vi "HB_ReadAIAllChannels.vi"(8 "error in (no error)":errorcluster, 11 "HBDeviceRef":T1) -> (0 "error out":errorcluster, 1 "All Channels Raw Values":u32[](array[numeric]) format="%012b", 2 "All Channels Scaled Values":dbl[](array[numeric]), 3 "HBDeviceRef":T1)   [LabVIEW 2016]
uses:
  <vilib>/Rock Robotics/WPI/SerialPort/WPI_SerialPortRef.ctl
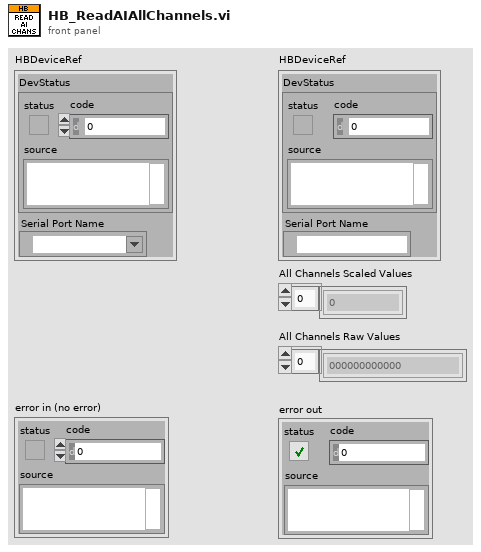
[diagram p1: front panel]
types:
  T1 = typedef "WPI_SerialPortRef.ctl" = cluster{"DevStatus":errorcluster, "Serial Port Name":refnum<visa-resource-name>}
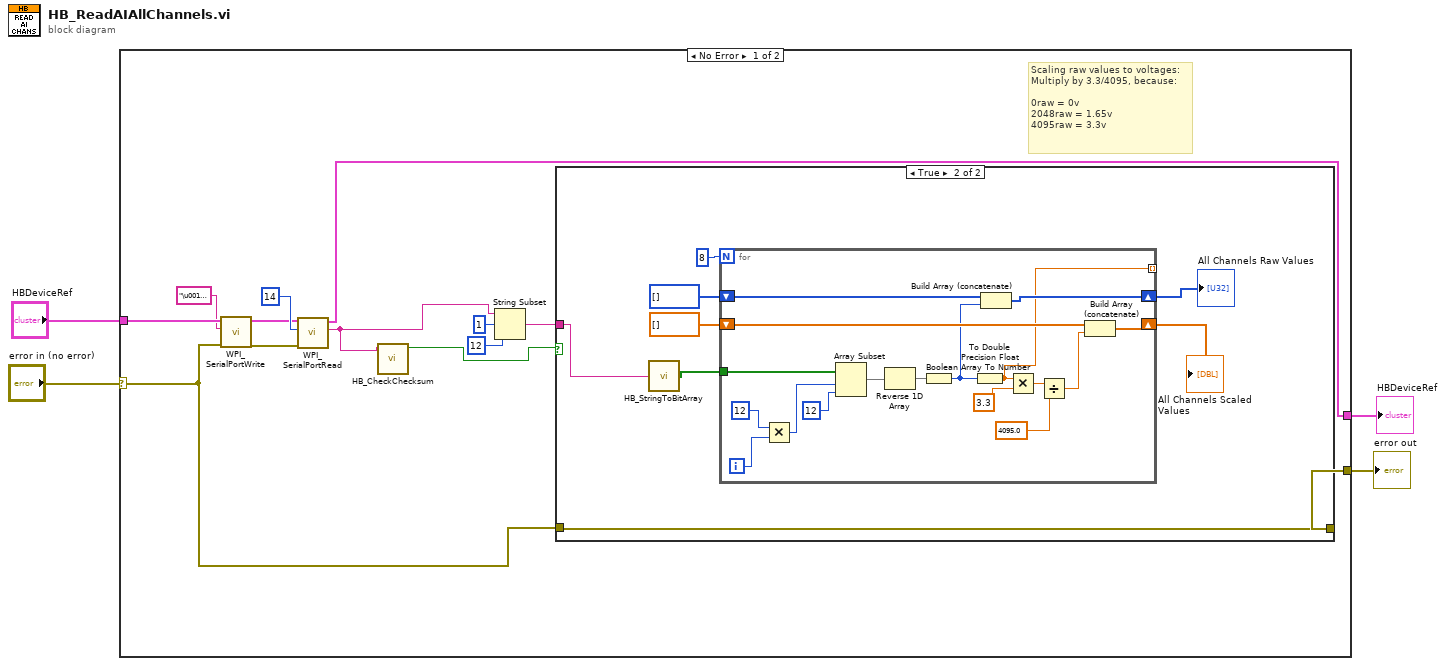
[diagram p0: block diagram]
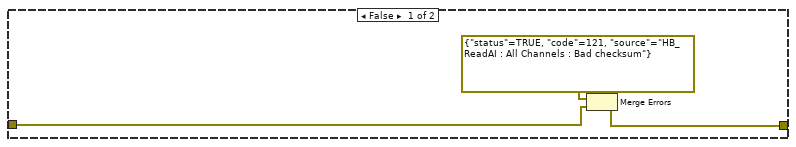
[diagram p2: hidden frame]
diagram:
  n1 = case shown="No Error" "error in (no error)" {
    selector: "error in (no error)" -> [w5 w46]
    tunnel: [w17 w46] -> w4
    tunnel: "HBDeviceRef" -> [w16 w47]
    tunnel: [w15 w47] -> w2
    frame No Error {
      # "Scaling raw values to voltages:\nMultiply by 3.3/4095, because:\n\n0raw = 0v\n2048raw = 1.65v\n4095raw = 3.3v"
      n2 = call <vilib>:"WPI_SerialPortWrite.vi"("error in (no error)"=w5, "Buffer"="\u0012\u0012", "SerialPortRef"=w16) -> ("error out"=w13:errorcluster, "SerialPortRef"=w12:T1)  [unwired: 6 in, 1 out]
      n3 = call <vilib>:"WPI_SerialPortRead.vi"("error in (no error)"=w13, "Num Bytes to Read"=u32 14, "SerialPortRef"=w12) -> ("Buffer"=w7:string, "SerialPortRef"=w15:T1)  [unwired: 6 in, 1 out]
      n4 = call <vilib>:"HB_CheckChecksum.vi"("String"=w7) -> ("Checksum Matches"=w6:bool)  [unwired: 9 in, 1 out]
      n5 = String Subset(string=w7, offset (0)=1, length (rest)=12 ("length (rest)")) -> (substring=w11:string)
      n6 = case shown="True" w6 {
        tunnel: w11 -> [_ w22]
        tunnel: w5 -> [w19 w28]
        tunnel: [w18 w28] -> w17
        frame False {
          n7 = Merge Errors(errorcluster {"status"=TRUE, "code"=121, "source"="HB_ReadAI : All Channels : Bad checksum"} ("error in"), w19) -> (w18:errorcluster)
        }
        frame True {
          n8 = call <vilib>:"HB_StringToBitArray.vi"("String"=w22) -> ("Bit Array"=w21:bool[])
          n9 = for {
            N: 8 -> [_]
            tunnel: w21 -> [w45]
            shift-right: [w41] -> w25
            shift-left: u32[] [] -> [w40]
            shift-right: [w36] -> w23
            shift-left: dbl[] [] -> [w35]
            tunnel: [w29] -> _ mode=indexing
            i -> [w44]
            n10 = Multiply(x=12, y=w44) -> (x*y=w42:i32)
            n11 = Array Subset(array=w45, index=w42, length=12) -> (w38:bool[])
            n12 = Reverse 1D Array(array=w38) -> (reversed array=w37:bool[])
            n13 = Boolean Array To Number(Boolean array=w37) -> (number=w30:u32)
            n14 = To Double Precision Float(number=w30) -> (double precision float=w29:dbl)
            n15 = Build Array (concatenate)(w40, w30) -> (w41:u32[])
            n16 = Multiply(x=w29, y=3.3) -> (x*y=w33:dbl)
            n17 = Divide(x=w33, y=4095.0) -> (x/y=w31:dbl)
            n18 = Build Array (concatenate)(w35, w31) -> (w36:dbl[])
          }
          "All Channels Raw Values" <- w25
          "All Channels Scaled Values" <- w23
        }
      }
    }
    frame Error {
    }
  }
  "error out" <- w4
  "HBDeviceRef" <- w2
